vi "Autonomous Independent.vi"() -> ()   [LabVIEW 2015]
doc: "This VI is called when autonomous begins, and will automatically be terminated when autonomous ends. You can carry out timed or sensor driven robot movement independently without needing to return to the caller."
uses:
  Type Defs/Auto Defense.ctl
  Type Defs/Auto Goal.ctl
  Type Defs/Auto Position.ctl
  Type Defs/Auto Goal Drive P4 M.ctl
  Type Defs/Auto Rough Terrain Cross.ctl
  Robot Global Data.vi
  <vilib>/addons/control/pid/pid.llb/PID (DBL).vi
  Type Defs/Auto Porticullis cross.ctl
  Type Defs/Auto Chival Cross.ctl
  Type Defs/Auto goal drive P5 R.ctl
  <instrlib>/navX Library v2/navX Library v2.lvlib
  Type Defs/Auto Goal Drive P4 R.ctl
  <vilib>/addons/control/pid/NI_PID_pid.lvlib
panel:
  in  "3nd fwd distance":dbl=4.0 format="%#_13g"
  in  "3nd fwd speed":dbl=-0.8 format="%#_13g"
  in  "Adjust Deadband Cross":dbl=0.5
  in  "Range Adjust":cluster{"output high":dbl, "output low":dbl}={"output high"=0.8, "output low"=-0.8} {"output low" format="%.2f"; "output high" format="%.2f"}
  in  "PID Adjust":T1={"proportional gain (Kc)"=0.2, "integral time (Ti, min)"=0.01, "derivative time (Td, min)"=0.0} {"derivative time (Td, min)" format="%.3f"; "integral time (Ti, min)" format="%.3f"; "proportional gain (Kc)" format="%.3f"}
  out "Yaw":dbl
  in  "Angle Setpoint":dbl format="%.2f"
  in  "PID Port 2":T1={"proportional gain (Kc)"=0.2, "integral time (Ti, min)"=0.01, "derivative time (Td, min)"=0.0} {"derivative time (Td, min)" format="%.3f"; "integral time (Ti, min)" format="%.3f"; "proportional gain (Kc)" format="%.3f"}
  in  "Range Port 2":cluster{"output high":dbl, "output low":dbl}={"output high"=0.8, "output low"=-0.8} {"output low" format="%.2f"; "output high" format="%.2f"}
  in  "Port 1st speed 2":dbl=-0.7
  in  "Port 1st Distance 2":dbl=4.5 format="%#_13g"
  in  "1st Turn Speed":dbl format="%#_13g"
  in  "1st turn angle":dbl format="%#_13g"
  in  "2nd fwd distance":dbl=4.0 format="%#_13g"
  in  "2nd fwd speed":dbl=-0.8 format="%#_13g"
  in  "2nd turn angle":dbl=-70.0 format="%#_13g"
  in  "2nd Turn Speed":dbl=0.7 format="%#_13g"
  in  "1st fwd speed":dbl=-0.75 format="%#_13g"
  in  "1st fwd distance":dbl=10.0 format="%#_13g"
  in  "RT Adjust Deadband":dbl=3.0
  in  "Range RT":cluster{"output high":dbl, "output low":dbl}={"output high"=0.8, "output low"=-0.8} {"output low" format="%.2f"; "output high" format="%.2f"}
  in  "PID RT":T1={"proportional gain (Kc)"=0.08, "integral time (Ti, min)"=0.01, "derivative time (Td, min)"=0.0} {"derivative time (Td, min)" format="%.3f"; "integral time (Ti, min)" format="%.3f"; "proportional gain (Kc)" format="%.3f"}
  in  "RT 1st Distance":dbl=9.5 format="%#_13g"
  in  "RT 2nd Speed":dbl=-0.9 format="%#_13g"
  in  "RT 1st speed":dbl=-0.9
  in  "RT speed error":dbl format="%#_13g"
  in  "RT shift speed distance":dbl=3.0 format="%#_13g"
  in  "2nd Distance Speed":dbl=-0.9 format="%#_13g"
  in  "Range Port":cluster{"output high":dbl, "output low":dbl}={"output high"=0.8, "output low"=-0.8} {"output low" format="%.2f"; "output high" format="%.2f"}
  in  "PID Port":T1={"proportional gain (Kc)"=0.2, "integral time (Ti, min)"=0.01, "derivative time (Td, min)"=0.0} {"derivative time (Td, min)" format="%.3f"; "integral time (Ti, min)" format="%.3f"; "proportional gain (Kc)" format="%.3f"}
  in  "Port 1st Distance":dbl=4.5 format="%#_13g"
  in  "Left Adjust":dbl
  in  "Right Adjust speed":dbl
  in  "Left Adjust speed":dbl
  in  "1st Distance Speed":dbl=-0.75 format="%#_13g"
  in  "Distance 1 Goal":dbl=11.5 format="%#_13g"
  in  "Chival Adjust Deadband":dbl=0.5
  in  "Range Chival":cluster{"output high":dbl, "output low":dbl}={"output high"=0.8, "output low"=-0.8} {"output low" format="%.2f"; "output high" format="%.2f"}
  in  "PID Chival":T1={"proportional gain (Kc)"=0.2, "integral time (Ti, min)"=0.01, "derivative time (Td, min)"=0.0} {"derivative time (Td, min)" format="%.3f"; "integral time (Ti, min)" format="%.3f"; "proportional gain (Kc)" format="%.3f"}
  in  "Arm Lift Distance":dbl=1.7 format="%#_13g"
  in  "Chival 2nd distance":dbl=6.0 format="%#_13g"
  in  "Chival Speed 2":dbl=-0.7
  in  "Chival Arm":dbl=100.0 format="%#_13g"
  in  "Chival Distance 1":dbl=3.0 format="%#_13g"
  in  "Chival speed":dbl=-0.7
  in  "Port 1st speed":dbl=-0.7
  in  "Distancia 1":dbl=3.0 format="%#_13g"
  in  "speed error":dbl=0.07 format="%#_13g"
  in  "velocidade 1":dbl
  in  "Adjust speed":dbl=-0.6 format="%#_13g"
  out "encoder":dbl
  out "x >= y?":bool
  out "Auto Angle":dbl
  out "erro":dbl
  in  "velocidade 2":dbl=0.7 format="%#_13g"
  in  "distancia 2":dbl=5.0 format="%#_13g"
  out "YRPHfH":T2
  # "Go to Right Goal from pos 5"
  # "Go to Middle goal from pos 4"
  # "Chival"
  # "Port"
  # "F lenta\nT Rapida"
  # "Rought Terrain"
  # "ramparts\nD 11"
  # "distancia speed\nrock wall 12 -1\n moat"
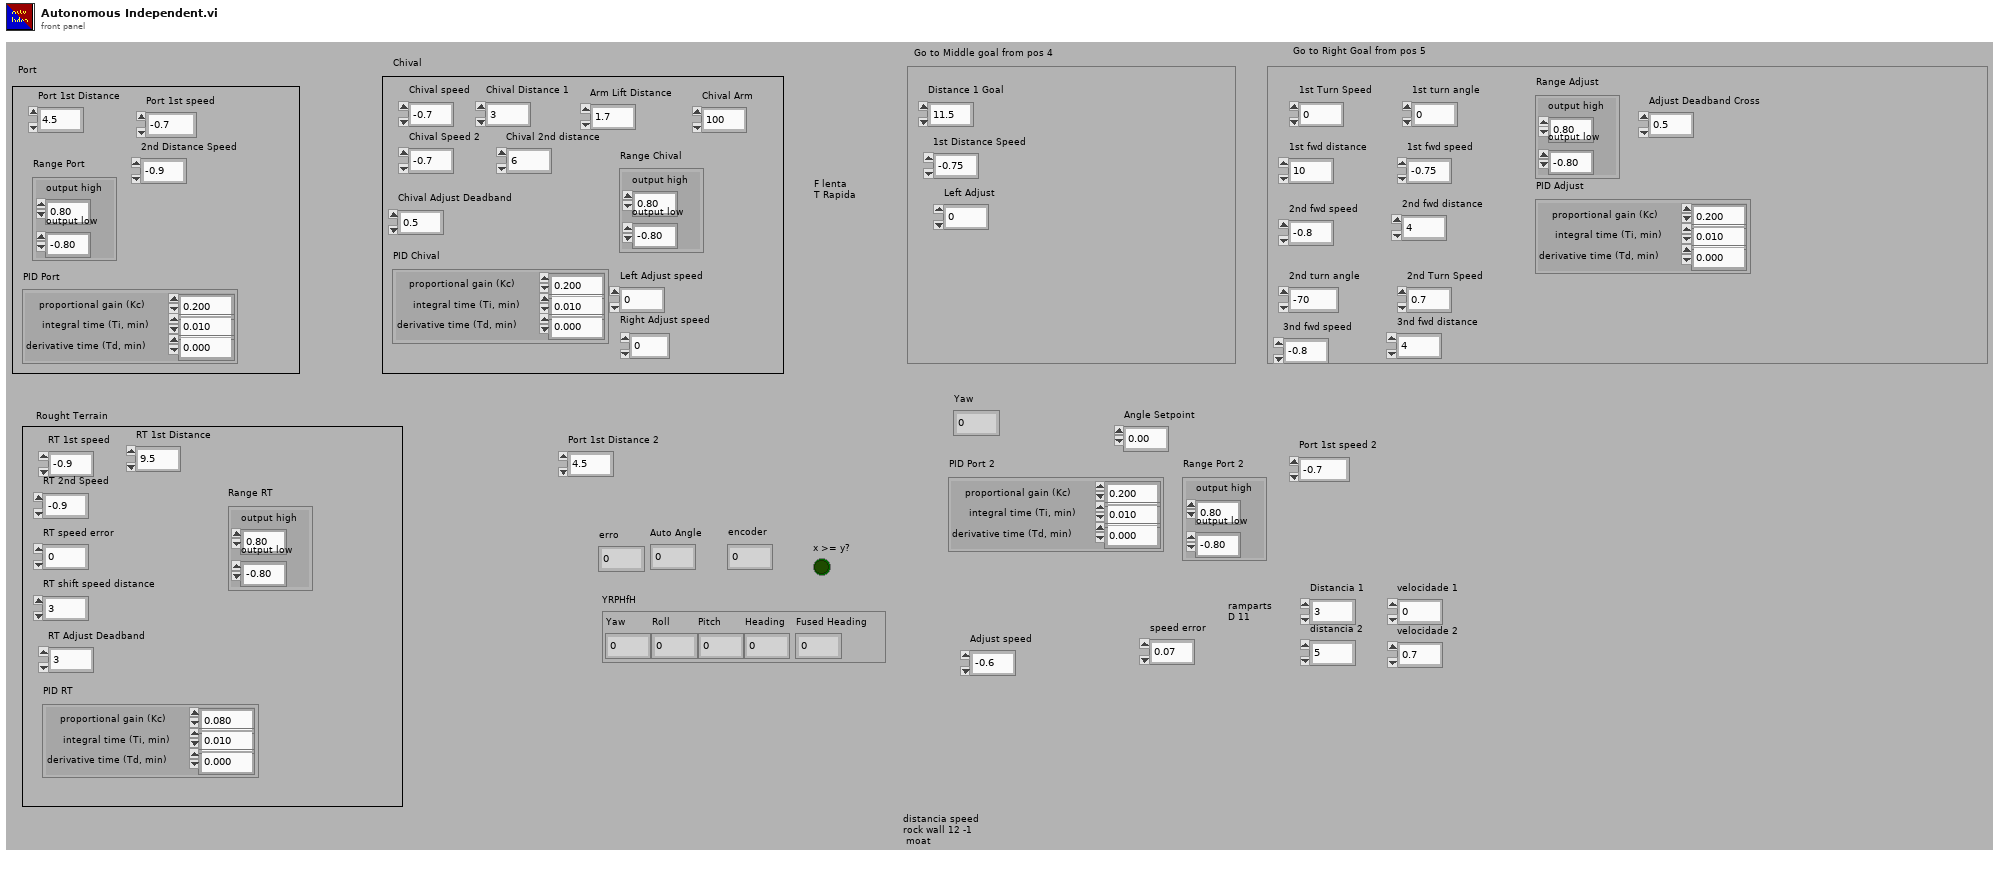
[diagram p1: front panel]
types:
  T1 = cluster{"proportional gain (Kc)":dbl, "integral time (Ti, min)":dbl, "derivative time (Td, min)":dbl}
  T2 = cluster{"Yaw":dbl, "Roll":dbl, "Pitch":dbl, "Heading":dbl, "Fused Heading":dbl}
  T3 = typedef "Auto Defense.ctl" = enum16{"Porticullis", "Chival de Frise", "Rough Terrain", "Rock Wall", "Ramparts", "Moat"}
  T4 = typedef "Auto Position.ctl" = enum16{"Pos 2", "Pos 3", "Pos 4", "Pos 5"}
  T5 = typedef "Auto Goal.ctl" = enum16{"Right Goal", "Left Goal", "Middle Goal"}
  T6 = typedef "Auto Goal Drive P4 R.ctl" = enum16{"Wait Defense Cross", "Turn Right", "Wait 1", "1st Forward", "Wait 2", "Turn Left", "Wait 3", "Adjust Left", "3rd Forward", "SHOOOOT", "Prepare Shoot"}
  T7 = typedef "Auto goal drive P5 R.ctl" = enum16{"Wait defense cross", "Adjust Right", "Wait 1", "1st Fwd", "Adjust Angle", "Wait 2", "2nd Fwd", "Turn Left", "Wait 3", "3nd Fwd", "Shoot"}
  T8 = typedef "Auto Goal Drive P4 M.ctl" = enum16{"Wait Defense Cross", "Prepare Shooter", "Go Fwd", "Shoot"}
  T9 = typedef "Auto Porticullis cross.ctl" = enum16{"Set Navx", "Go Fwd", "Wait 1", "Cross Porticullis", "Get Navx", "Adjust angle", "Wait 2", "Finish"}
  T10 = typedef "Auto Chival Cross.ctl" = enum16{"Set NavX", "Go Fwd", "Lower Arm", "Slow Fwd", "Get NavX", "Adjust Angle", "Wait", "Finish"}
  T11 = typedef "Auto Rough Terrain Cross.ctl" = enum16{"Set NavX", "Go Fwd", "Get Navx", "Correct Angle", "Wait", "Go to Goal"}
  T12 = enum16{"Set NavX", "Go Fwd", "Get Navx", "Correct Angle", "Go to Goal"}
  T13 = typedef "navX Library v2.lvlib/Z900_navX_DeviceTypeDef.ctl" = cluster{"Interface":cluster{"Protocol":T14, "Update Rate (4Hz-60Hz)":u8, "navX Open TypeDef":variant}, "Notify Packet":refnum<notifier>, "Loop VI Refnum":refnum<vi>, "Ready to Close Occurrence Refnum":refnum<k4>}
  T14 = typedef "navX Library v2.lvlib/Z900_navX_ProtocolTypeDef.ctl" = enum16{"SERIAL", "I2C", "SPI"}
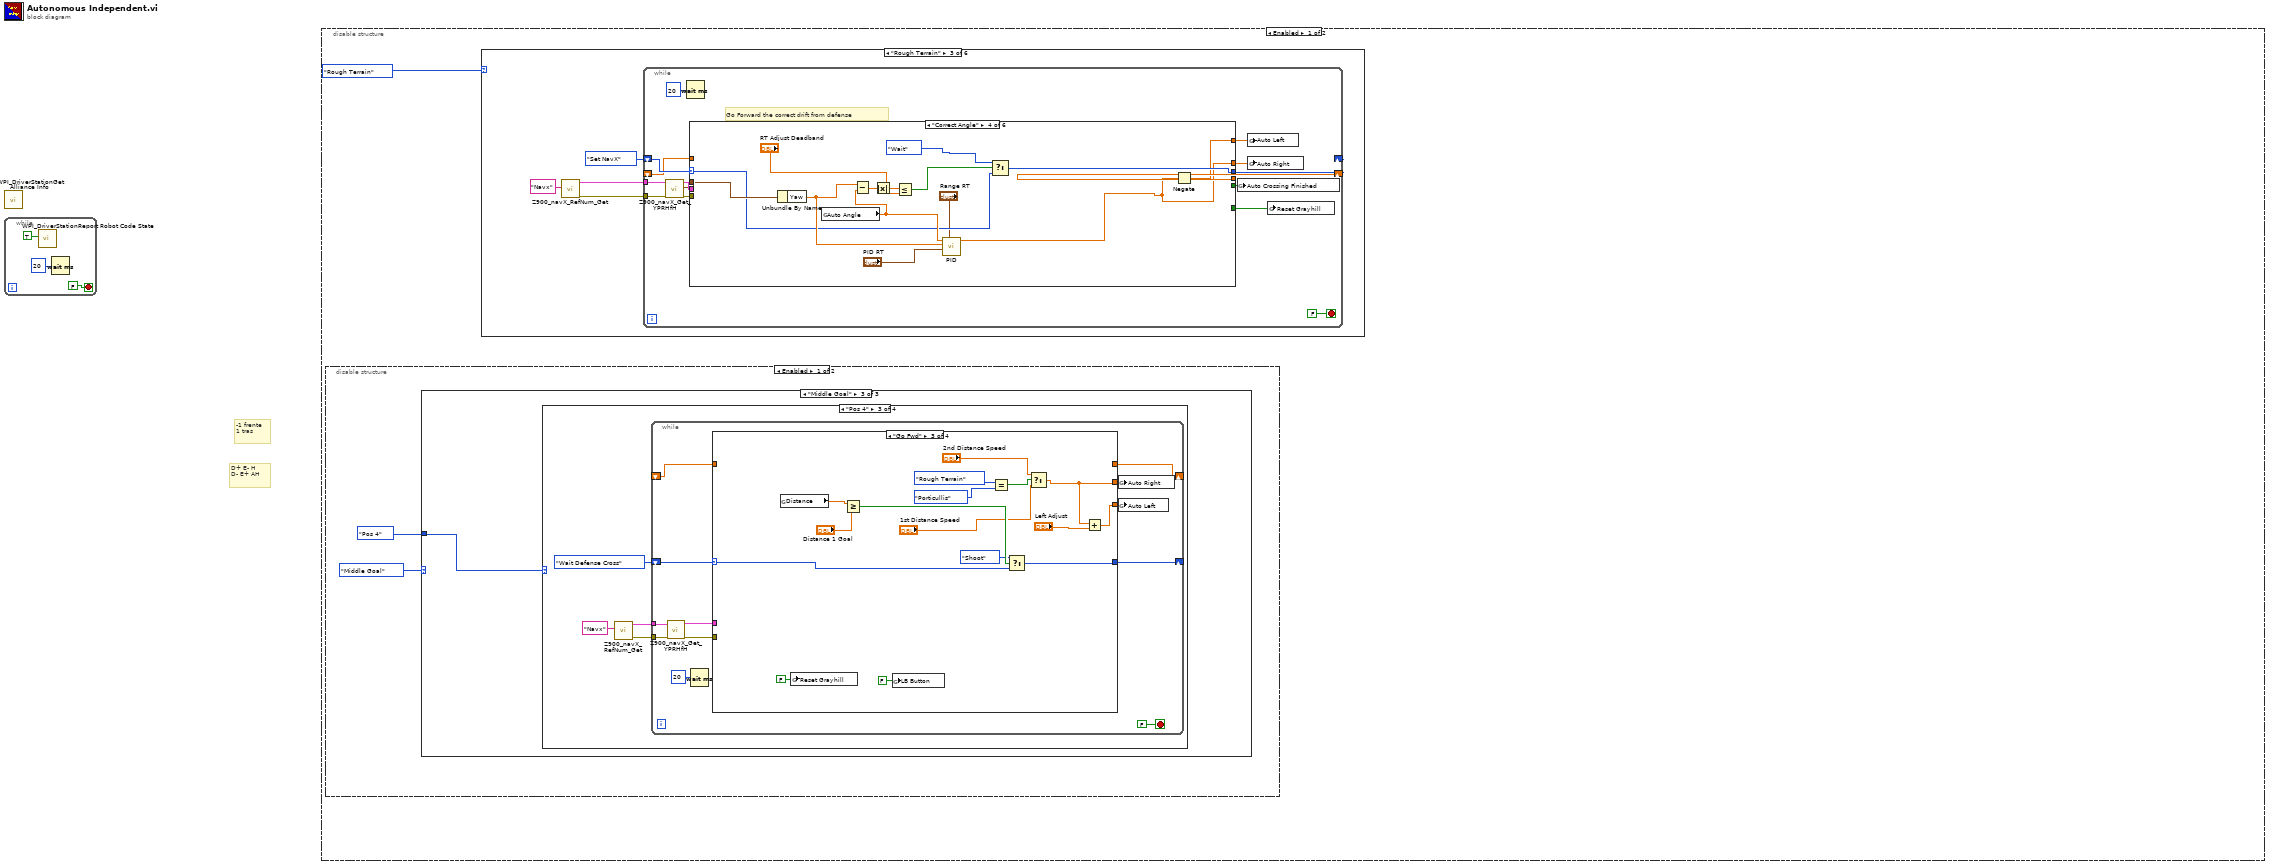
[diagram p0: block diagram]
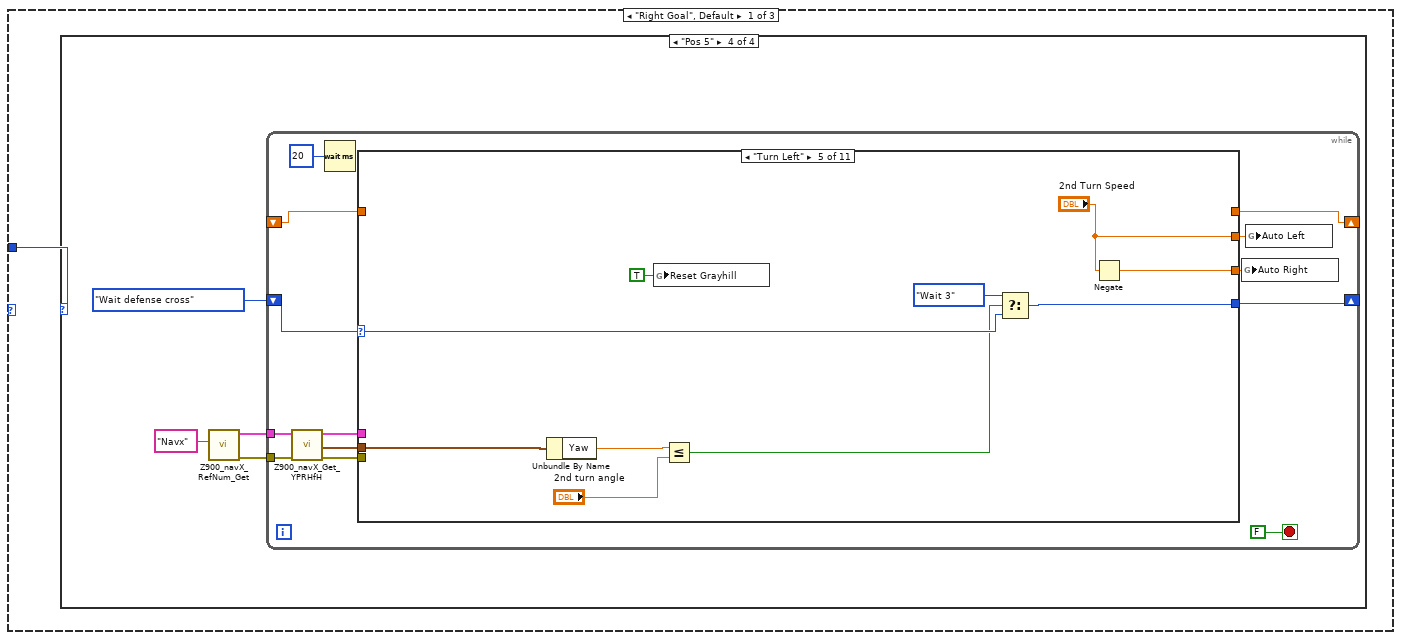
[diagram p2: hidden frame]
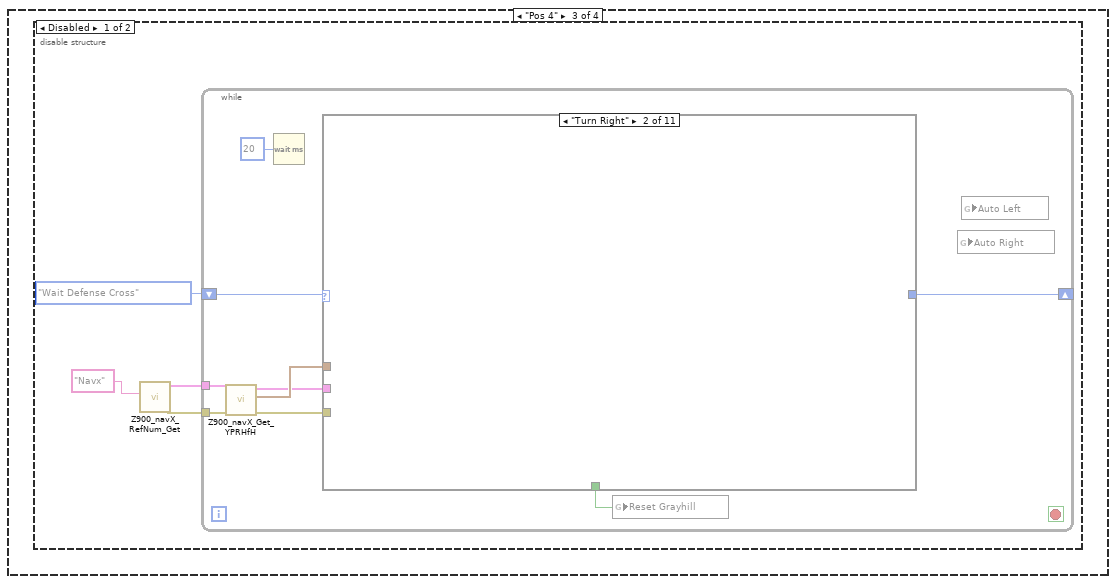
[diagram p5: hidden frame]
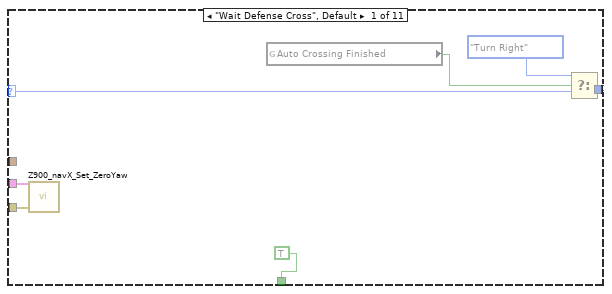
[diagram p6: hidden frame]
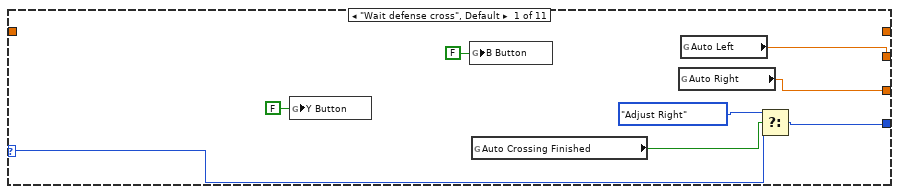
[diagram p17: hidden frame]
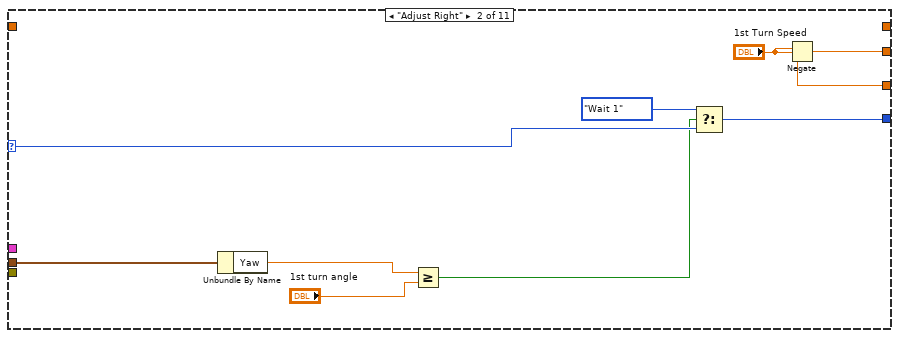
[diagram p18: hidden frame]
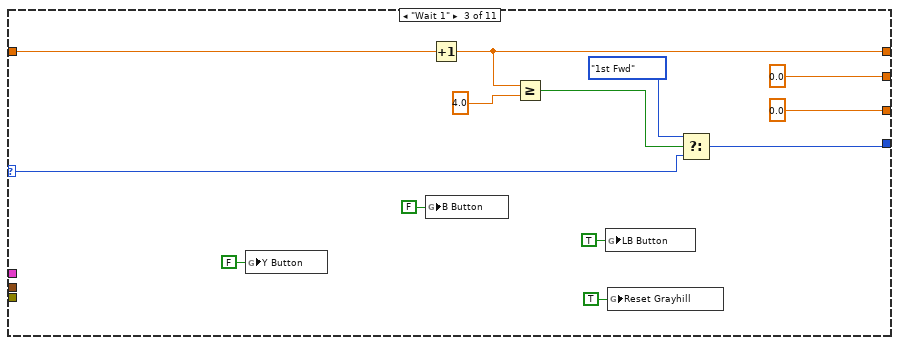
[diagram p19: hidden frame]
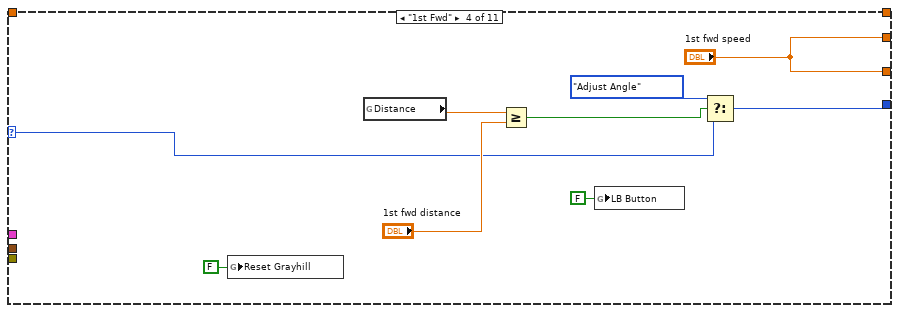
[diagram p20: hidden frame]
diagram:
  # "D+ E- H\nD- E+ AH"
  # "-1 frente\n1 tras"
  n1 = call <vilib>:"WPI_DriverStationGet Alliance Info.vi"() -> ()  [unwired: 12 out]
  n2 = while {
    stop <- FALSE stop-if-true
    n3 = call <vilib>:"WPI_DriverStationReport Robot Code State.vi"("Autonomous"=TRUE) -> ()  [unwired: 10 in, 1 out]
    n4 = Wait (ms)(milliseconds to wait=u32 20) -> ()  [unwired: 1 out]
  }
  n5 = disable-structure shown="Enabled" {
    frame Enabled {
      n6 = disable-structure shown="Enabled" {
        frame Enabled {
          n7 = case shown="\"Middle Goal\"" Auto_Goal."Middle Goal" {
            tunnel: Auto_Position."Pos 4" -> [w7 w150 w151]
            frame "Right Goal", Default {
              n8 = case shown="\"Pos 5\"" w7 {
                frame "Pos 2", Default {
                }
                frame "Pos 3" {
                }
                frame "Pos 4" {
                  n9 = disable-structure shown="Disabled" {
                    frame Disabled {
                      n10 = call <instrlib>:"Z900_navX_RefNum_Get.vi"("refnum name"="Navx") -> ("error out"=w8:errorcluster, "navX Device"=w9:T13)  [unwired: 9 in]
                      n11 = while {
                        shift-right: [w14] -> _
                        shift-left: Auto_Goal_Drive_P4_R."Wait Defense Cross" -> [w20]
                        tunnel: w9 -> [w19]
                        tunnel: w8 -> [w18]
                        stop <- _ stop-if-true
                        n12 = call <instrlib>:"Z900_navX_Get_YPRHfH.vi"("error in (no error)"=w18, "navX Device"=w19) -> ("error out"=w15:errorcluster, "YRPHfH"=w17:T2, "navX Device"=w16:T13)  [unwired: 6 in, 1 out]
                        n13 = Wait (ms)(milliseconds to wait=u32 20) -> ()  [unwired: 1 out]
                        n14 = case shown="\"Turn Right\"" w20 {
                          selector: w20 -> [w24 _ _ _ _ _ _ _ _ _ _]
                          tunnel: w17 -> [_ _ _ _ _ _ _ _ _ _ _]
                          tunnel: w16 -> [w27 _ _ _ _ _ _ _ _ _ _]
                          tunnel: w15 -> [w26 _ _ _ _ _ _ _ _ _ _]
                          tunnel: [w25 _ _ _ _ _ _ _ _ _ _] -> w14
                          tunnel: [TRUE _ _ _ _ _ _ _ _ _ _] -> w12
                          frame "Wait Defense Cross", Default {
                            n15 = call <instrlib>:"Z900_navX_Set_ZeroYaw.vi"("error in (no error)"=w26, "navX Device"=w27) -> ()  [unwired: 8 in, 2 out]
                            n16 = global read "Robot Global Data.vi" "Auto Crossing Finished"() -> (w22:bool)
                            n17 = Select(t=Auto_Goal_Drive_P4_R."Turn Right", s=w22, f=w24) -> (s? t:f=w25:T6)
                          }
                          frame "Turn Right" {
                          }
                          frame "Wait 1" {
                          }
                          frame "1st Forward" {
                          }
                          frame "Wait 2" {
                          }
                          frame "Turn Left" {
                          }
                          frame "Wait 3" {
                          }
                          frame "Adjust Left" {
                          }
                          frame "3rd Forward" {
                          }
                          frame "SHOOOOT" {
                          }
                          frame "Prepare Shoot" {
                          }
                        }
                        n18 = global write "Robot Global Data.vi" "Reset Grayhill"(w12) -> ()
                        n19 = global read "Robot Global Data.vi" "Auto Right"() -> ()  [unwired: 1 in]
                        n20 = global read "Robot Global Data.vi" "Auto Left"() -> ()  [unwired: 1 in]
                      }
                    }
                    frame Enabled {
                    }
                  }
                }
                frame "Pos 5" {
                  n21 = call <instrlib>:"Z900_navX_RefNum_Get.vi"("refnum name"="Navx") -> ("error out"=w28:errorcluster, "navX Device"=w29:T13)  [unwired: 9 in]
                  n22 = while {
                    shift-right: [w42] -> _
                    shift-left: Auto_goal_drive_P5_R."Wait defense cross" -> [w44]
                    tunnel: w29 -> [w40]
                    tunnel: w28 -> [w39]
                    shift-right: [w32] -> _
                    shift-left: _ -> [w33]
                    stop <- FALSE stop-if-true
                    n23 = call <instrlib>:"Z900_navX_Get_YPRHfH.vi"("error in (no error)"=w39, "navX Device"=w40) -> ("error out"=w34:errorcluster, "YRPHfH"=w38:T2, "navX Device"=w35:T13)  [unwired: 6 in, 1 out]
                    n24 = Wait (ms)(milliseconds to wait=u32 20) -> ()  [unwired: 1 out]
                    n25 = case shown="\"Turn Left\"" w44 {
                      selector: w44 -> [w51 w59 w70 w76 w92 _ w103 w112 w119 w131 w145]
                      tunnel: [w52 w60 w71 w78 w93 Auto_goal_drive_P5_R."Shoot" w104 w114 w120 w130 w144] -> w42
                      tunnel: w38 -> [_ w61 _ _ w91 _ _ _ _ w132 _]
                      tunnel: [w48 w54 0.0 "1st fwd speed" "2nd Turn Speed" w99 "2nd fwd speed" 0.0 "3nd fwd speed" w128 0.0] -> w37
                      tunnel: [w47 "1st Turn Speed" 0.0 "1st fwd speed" w85 w99 "2nd fwd speed" 0.0 "3nd fwd speed" w127 0.0] -> w36
                      tunnel: w35 -> [_ _ _ _ _ _ _ _ _ _ _]
                      tunnel: w34 -> [_ _ _ _ _ _ _ _ _ _ _]
                      tunnel: w33 -> [_ _ w69 _ _ w97 _ w111 _ _ w146]
                      tunnel: [_ _ w68 _ _ w96 _ w113 _ _ w141] -> w32
                      frame "Wait defense cross", Default {
                        n26 = global write "Robot Global Data.vi" "Y Button"(FALSE ("Y Button")) -> ()
                        n27 = global write "Robot Global Data.vi" "B Button"(FALSE ("B Button")) -> ()
                        n28 = global read "Robot Global Data.vi" "Auto Crossing Finished"() -> (w49:bool)
                        n29 = global read "Robot Global Data.vi" "Auto Right"() -> (w47:dbl)
                        n30 = global read "Robot Global Data.vi" "Auto Left"() -> (w48:dbl)
                        n31 = Select(t=Auto_goal_drive_P5_R."Adjust Right", s=w49, f=w51) -> (s? t:f=w52:T7)
                      }
                      frame "Adjust Right" {
                        n32 = Unbundle By Name(w61) -> ("Yaw"=w58:dbl)
                        n33 = Greater Or Equal?(x=w58, y="1st turn angle") -> (x >= y?=w56:bool)
                        n34 = Select(t=Auto_goal_drive_P5_R."Wait 1", s=w56, f=w59) -> (s? t:f=w60:T7)
                        n35 = Negate(x="1st Turn Speed") -> (-x=w54:dbl)
                      }
                      frame "Wait 1" {
                        n36 = global write "Robot Global Data.vi" "Y Button"(FALSE ("Y Button")) -> ()
                        n37 = global write "Robot Global Data.vi" "B Button"(FALSE ("B Button")) -> ()
                        n38 = Increment(x=w69) -> (x+1=w68:dbl)
                        n39 = Greater Or Equal?(x=w68, y=4.0) -> (x >= y?=w67:bool)
                        n40 = global write "Robot Global Data.vi" "LB Button"(TRUE ("LB Button")) -> ()
                        n41 = global write "Robot Global Data.vi" "Reset Grayhill"(TRUE ("Reset Grayhill")) -> ()
                        n42 = Select(t=Auto_goal_drive_P5_R."1st Fwd", s=w67, f=w70) -> (s? t:f=w71:T7)
                      }
                      frame "1st Fwd" {
                        n43 = global write "Robot Global Data.vi" "Reset Grayhill"(FALSE ("Reset Grayhill")) -> ()
                        n44 = global read "Robot Global Data.vi" "Distance"() -> (w80:dbl)
                        n45 = Greater Or Equal?(x=w80, y="1st fwd distance") -> (x >= y?=w77:bool)
                        n46 = global write "Robot Global Data.vi" "LB Button"(FALSE ("LB Button")) -> ()
                        n47 = Select(t=Auto_goal_drive_P5_R."Adjust Angle", s=w77, f=w76) -> (s? t:f=w78:T7)
                      }
                      frame "Turn Left" {
                        n48 = Unbundle By Name(w91) -> ("Yaw"=w89:dbl)
                        n49 = global write "Robot Global Data.vi" "Reset Grayhill"(TRUE ("Reset Grayhill")) -> ()
                        n50 = Less Or Equal?(x=w89, y="2nd turn angle") -> (x <= y?=w87:bool)
                        n51 = Select(t=Auto_goal_drive_P5_R."Wait 3", s=w87, f=w92) -> (s? t:f=w93:T7)
                        n52 = Negate(x="2nd Turn Speed") -> (-x=w85:dbl)
                      }
                      frame "Shoot" {
                        w99 = -0.3
                        n53 = Increment(x=w97) -> (x+1=w96:dbl)
                        n54 = Greater Or Equal?(x=w96, y=20.0) -> (x >= y?=w94:bool)
                        n55 = global write "Robot Global Data.vi" "RB Trigger"(w94) -> ()
                      }
                      frame "2nd Fwd" {
                        n56 = global read "Robot Global Data.vi" "Distance"() -> (w107:dbl)
                        n57 = Greater Or Equal?(x=w107, y="2nd fwd distance") -> (x >= y?=w102:bool)
                        n58 = global write "Robot Global Data.vi" "Reset Grayhill"(FALSE ("Reset Grayhill")) -> ()
                        n59 = Select(t=Auto_goal_drive_P5_R."Turn Left", s=w102, f=w103) -> (s? t:f=w104:T7)
                      }
                      frame "Wait 3" {
                        n60 = Increment(x=w111) -> (x+1=w113:dbl)
                        n61 = Greater Or Equal?(x=w113, y=4.0) -> (x >= y?=w117:bool)
                        n62 = global write "Robot Global Data.vi" "Reset Grayhill"(TRUE ("Reset Grayhill")) -> ()
                        n63 = Select(t=Auto_goal_drive_P5_R."3nd Fwd", s=w117, f=w112) -> (s? t:f=w114:T7)
                      }
                      frame "3nd Fwd" {
                        n64 = global read "Robot Global Data.vi" "Distance"() -> (w125:dbl)
                        n65 = Greater Or Equal?(x=w125, y="3nd fwd distance") -> (x >= y?=w123:bool)
                        n66 = Select(t=Auto_goal_drive_P5_R."Shoot", s=w123, f=w119) -> (s? t:f=w120:T7)
                        n67 = global write "Robot Global Data.vi" "Reset Grayhill"(FALSE ("Reset Grayhill")) -> ()
                      }
                      frame "Adjust Angle" {
                        n68 = Unbundle By Name(w132) -> ("Yaw"=w138:dbl)
                        n69 = global read "Robot Global Data.vi" "Auto Angle"() -> (w137:dbl)
                        n70 = Subtract(x=w138, y=w137) -> (x-y=w136:dbl)
                        n71 = Absolute Value(x=w136) -> (abs(x)=w135:dbl)
                        n72 = Less Or Equal?(x=w135, y="Adjust Deadband Cross") -> (x <= y?=w133:bool)
                        n73 = call-poly <vilib>:"PID.vi"("output range"="Range Adjust", "PID gains"="PID Adjust", "process variable"=w138, "setpoint"=w137) -> ("output"=w127:dbl)  [unwired: 6 in, 1 out]
                        n74 = Select(t=Auto_goal_drive_P5_R."Wait 2", s=w133, f=w131) -> (s? t:f=w130:T7)
                        n75 = Negate(x=w127) -> (-x=w128:dbl)
                      }
                      frame "Wait 2" {
                        n76 = global write "Robot Global Data.vi" "Reset Grayhill"(TRUE ("Reset Grayhill")) -> ()
                        n77 = Increment(x=w146) -> (x+1=w141:dbl)
                        n78 = Greater Or Equal?(x=w141, y=4.0) -> (x >= y?=w149:bool)
                        n79 = Select(t=Auto_goal_drive_P5_R."2nd Fwd", s=w149, f=w145) -> (s? t:f=w144:T7)
                      }
                    }
                    n80 = global write "Robot Global Data.vi" "Auto Right"(w36) -> ()
                    n81 = global write "Robot Global Data.vi" "Auto Left"(w37) -> ()
                  }
                }
              }
            }
            frame "Left Goal" {
              n82 = case shown="\"Pos 3\"" w150 {
                frame "Pos 2", Default {
                }
                frame "Pos 3" {
                }
                frame "Pos 4" {
                }
                frame "Pos 5" {
                }
              }
            }
            frame "Middle Goal" {
              n83 = case shown="\"Pos 4\"" w151 {
                frame "Pos 2", Default {
                }
                frame "Pos 3" {
                }
                frame "Pos 4" {
                  n84 = call <instrlib>:"Z900_navX_RefNum_Get.vi"("refnum name"="Navx") -> ("error out"=w152:errorcluster, "navX Device"=w153:T13)  [unwired: 9 in]
                  n85 = while {
                    shift-right: [w164] -> _
                    shift-left: Auto_Goal_Drive_P4_M."Wait Defense Cross" -> [w167]
                    tunnel: w153 -> [w163]
                    tunnel: w152 -> [w162]
                    shift-right: [w157] -> _
                    shift-left: _ -> [w156]
                    stop <- FALSE stop-if-true
                    n86 = call <instrlib>:"Z900_navX_Get_YPRHfH.vi"("error in (no error)"=w162, "navX Device"=w163) -> ("error out"=w160:errorcluster, "navX Device"=w161:T13)  [unwired: 6 in, 2 out]
                    n87 = Wait (ms)(milliseconds to wait=u32 20) -> ()  [unwired: 1 out]
                    n88 = case shown="\"Go Fwd\"" w167 {
                      selector: w167 -> [w173 w176 w197 _]
                      tunnel: [w172 w177 w198 Auto_Goal_Drive_P4_M."Shoot"] -> w164
                      tunnel: w161 -> [_ _ _ _]
                      tunnel: w160 -> [_ _ _ _]
                      tunnel: [w170 w182 w191 w208] -> w159
                      tunnel: [w169 w182 w188 w208] -> w158
                      tunnel: [_ w180 _ w210] -> w157
                      tunnel: w156 -> [_ w181 _ w211]
                      frame "Wait Defense Cross", Default {
                        w168 = FALSE
                        n89 = global read "Robot Global Data.vi" "Auto Crossing Finished"() -> (w174:bool)
                        n90 = global write "Robot Global Data.vi" "B Button"(w168) -> ()
                        n91 = global write "Robot Global Data.vi" "Y Button"(w168) -> ()
                        n92 = Select(t=Auto_Goal_Drive_P4_M."Prepare Shooter", s=w174, f=w173) -> (s? t:f=w172:T8)
                        n93 = global read "Robot Global Data.vi" "Auto Right"() -> (w169:dbl)
                        n94 = global read "Robot Global Data.vi" "Auto Left"() -> (w170:dbl)
                      }
                      frame "Prepare Shooter" {
                        w182 = 0.0 ("Auto Right")
                        n95 = global write "Robot Global Data.vi" "Reset Grayhill"(TRUE ("Reset Grayhill")) -> ()
                        n96 = Increment(x=w181) -> (x+1=w180:dbl)
                        n97 = global write "Robot Global Data.vi" "LB Button"(TRUE ("LB Button")) -> ()
                        n98 = Greater Or Equal?(x=w180, y=5.0) -> (x >= y?=w175:bool)
                        n99 = Select(t=Auto_Goal_Drive_P4_M."Go Fwd", s=w175, f=w176) -> (s? t:f=w177:T8)
                      }
                      frame "Go Fwd" {
                        n100 = global read "Robot Global Data.vi" "Distance"() -> (w196:dbl)
                        n101 = global write "Robot Global Data.vi" "Reset Grayhill"(FALSE ("Reset Grayhill")) -> ()
                        n102 = Greater Or Equal?(x=w196, y="Distance 1 Goal") -> (x >= y?=w194:bool)
                        n103 = global write "Robot Global Data.vi" "LB Button"(FALSE ("LB Button")) -> ()
                        n104 = Equal?(x=Auto_Defense."Rough Terrain", y=Auto_Defense."Porticullis") -> (x = y?=w187:bool)
                        n105 = Select(t=Auto_Goal_Drive_P4_M."Shoot", s=w194, f=w197) -> (s? t:f=w198:T8)
                        n106 = Select(t="2nd Distance Speed", s=w187, f="1st Distance Speed") -> (s? t:f=w188:dbl)
                        n107 = Add(x=w188, y="Left Adjust") -> (x+y=w191:dbl)
                      }
                      frame "Shoot" {
                        w208 = -0.6 ("Auto Right")
                        # "Alterar para chamada da dashboard"
                        n108 = Increment(x=w211) -> (x+1=w210:dbl)
                        n109 = Equal?(x=Auto_Defense."Rough Terrain", y=Auto_Defense."Porticullis") -> (x = y?=w203:bool)
                        n110 = Select(t=80.0 ("y"), s=w203, f=40.0) -> (s? t:f=w204:dbl)
                        n111 = Greater Or Equal?(x=w210, y=w204) -> (x >= y?=w207:bool)
                        n112 = global write "Robot Global Data.vi" "RB Trigger"(w207) -> ()
                      }
                    }
                    n113 = global write "Robot Global Data.vi" "Auto Right"(w158) -> ()
                    n114 = global write "Robot Global Data.vi" "Auto Left"(w159) -> ()
                  }
                }
                frame "Pos 5" {
                }
              }
            }
          }
        }
        frame Disabled {
        }
      }
      n115 = case shown="\"Rough Terrain\"" Auto_Defense."Rough Terrain" {
        frame "Porticullis", Default {
          n116 = disable-structure shown="Enabled" {
            frame Enabled {
              n117 = call <instrlib>:"Z900_navX_RefNum_Get.vi"("refnum name"="Navx") -> ("error out"=w213:errorcluster, "navX Device"=w214:T13)  [unwired: 9 in]
              n118 = while {
                shift-right: [w231] -> _
                shift-left: Auto_Porticullis_cross."Set Navx" -> [w232]
                tunnel: w214 -> [w230]
                tunnel: w213 -> [w229]
                shift-right: [w225] -> _
                shift-left: _ -> [w224]
                shift-right: [w216] -> _
                shift-left: _ -> [w217]
                stop <- FALSE stop-if-true
                n119 = call <instrlib>:"Z900_navX_Get_YPRHfH.vi"("error in (no error)"=w229, "navX Device"=w230) -> ("error out"=w228:errorcluster, "YRPHfH"=w226:T2, "navX Device"=w227:T13)  [unwired: 6 in, 1 out]
                n120 = Wait (ms)(milliseconds to wait=u32 20) -> ()  [unwired: 1 out]
                n121 = case shown="\"Set Navx\", Default" w232 {
                  selector: w232 -> [w241 w248 w257 w268 w277 w291 _ w308]
                  tunnel: [w242 w250 w258 w269 w276 w290 Auto_Porticullis_cross."Finish" w310] -> w231
                  tunnel: w228 -> [w240 _ _ _ _ _ _ _]
                  tunnel: w227 -> [w239 _ _ _ _ _ _ _]
                  tunnel: w226 -> [w238 _ _ _ w278 w292 _ _]
                  tunnel: [w237 _ w259 _ w279 _ _ _] -> w225
                  tunnel: w224 -> [w236 _ w264 _ w280 _ _ _]
                  tunnel: [w235 "Port 1st speed" 0.0 ("Port speed") 0.0 ("Port speed") w274 w286 w301 w312] -> w223
                  tunnel: [w235 "Port 1st speed" 0.0 ("Port speed") 0.0 ("Port speed") w274 w287 w302 w312] -> w222
                  tunnel: [TRUE _ TRUE w265 TRUE _ w300 _] -> w221
                  tunnel: [_ _ _ _ _ _ TRUE _] -> w219
                  tunnel: w217 -> [_ _ _ _ _ _ _ w311]
                  tunnel: [_ _ _ _ _ _ _ w307] -> w216
                  frame "Set Navx", Default {
                    w235 = 0.0
                    n122 = call <instrlib>:"Z900_navX_Set_ZeroYaw.vi"("error in (no error)"=w240, "navX Device"=w239) -> ()  [unwired: 8 in, 2 out]
                    n123 = Unbundle By Name(w238) -> ("Yaw"=w245:dbl)
                    n124 = Increment(x=w236) -> (x+1=w237:dbl)
                    n125 = global write "Robot Global Data.vi" "Auto Angle"(w245) -> ()
                    n126 = Greater Or Equal?(x=w237, y=3.0) -> (x >= y?=w243:bool)
                    n127 = Select(t=Auto_Porticullis_cross."Go Fwd", s=w243, f=w241) -> (s? t:f=w242:T9)
                  }
                  frame "Go Fwd" {
                    n128 = global write "Robot Global Data.vi" "B Button"(TRUE ("B Button")) -> ()
                    n129 = global read "Robot Global Data.vi" "Distance"() -> (w252:dbl)
                    n130 = Greater Or Equal?(x=w252, y="Port 1st Distance") -> (x >= y?=w249:bool)
                    n131 = Select(t=Auto_Porticullis_cross."Cross Porticullis", s=w249, f=w248) -> (s? t:f=w250:T9)
                  }
                  frame "Wait 1" {
                    n132 = global write "Robot Global Data.vi" "B Button"(FALSE ("B Button")) -> ()
                    n133 = Increment(x=w264) -> (x+1=w259:dbl)
                    n134 = Greater Or Equal?(x=w259, y=30.0) -> (x >= y?=w260:bool)
                    n135 = Select(t=Auto_Porticullis_cross."Cross Porticullis", s=w260, f=w257) -> (s? t:f=w258:T9)
                  }
                  frame "Cross Porticullis" {
                    n136 = global write "Robot Global Data.vi" "Start Button"(TRUE ("Start Button")) -> ()
                    n137 = global read "Robot Global Data.vi" "Finished Porticullis crossing"() -> (w267:bool)
                    n138 = Select(t=Auto_Porticullis_cross."Get Navx", s=w267, f=w268) -> (s? t:f=w269:T9)
                    n139 = global read "Robot Global Data.vi" "Reset Grayhill"() -> (w265:bool)
                  }
                  frame "Get Navx" {
                    w274 = 0.0
                    n140 = Unbundle By Name(w278) -> ("Yaw"=w285:dbl)
                    n141 = global read "Robot Global Data.vi" "Auto Angle"() -> (w284:dbl)
                    n142 = Increment(x=w280) -> (x+1=w279:dbl)
                    n143 = Greater Or Equal?(x=w279, y=3.0) -> (x >= y?=w281:bool)
                    n144 = Subtract(x=w285, y=w284) -> (x-y=w282:dbl)
                    n145 = Select(t=Auto_Porticullis_cross."Adjust angle", s=w281, f=w277) -> (s? t:f=w276:T9)
                    n146 = global write "Robot Global Data.vi" "Auto Angle error"(w282) -> ()
                  }
                  frame "Adjust angle" {
                    n147 = Unbundle By Name(w292) -> ("Yaw"=w297:dbl)
                    n148 = global read "Robot Global Data.vi" "Auto Angle"() -> (w296:dbl)
                    n149 = Subtract(x=w297, y=w296) -> (x-y=w295:dbl)
                    n150 = Absolute Value(x=w295) -> (abs(x)=w294:dbl)
                    n151 = Less Or Equal?(x=w294, y=3.0) -> (x <= y?=w293:bool)
                    n152 = call-poly <vilib>:"PID.vi"("output range"="Range Port", "PID gains"="PID Port", "process variable"=w297, "setpoint"=w296) -> ("output"=w287:dbl)  [unwired: 6 in, 1 out]
                    n153 = Select(t=Auto_Porticullis_cross."Wait 2", s=w293, f=w291) -> (s? t:f=w290:T9)
                    n154 = Negate(x=w287) -> (-x=w286:dbl)
                  }
                  frame "Finish" {
                    n155 = global read "Robot Global Data.vi" "Reset Grayhill"() -> (w300:bool)
                    n156 = global read "Robot Global Data.vi" "Auto Right"() -> (w302:dbl)
                    n157 = global read "Robot Global Data.vi" "Auto Left"() -> (w301:dbl)
                  }
                  frame "Wait 2" {
                    w312 = 0.0 ("Auto Right")
                    n158 = Increment(x=w311) -> (x+1=w307:dbl)
                    n159 = Greater Or Equal?(x=w307, y=25.0) -> (x >= y?=w305:bool)
                    n160 = Select(t=Auto_Porticullis_cross."Finish", s=w305, f=w308) -> (s? t:f=w310:T9)
                  }
                }
                n161 = global write "Robot Global Data.vi" "Auto Right"(w222) -> ()
                n162 = global write "Robot Global Data.vi" "Auto Left"(w223) -> ()
                n163 = global write "Robot Global Data.vi" "Reset Grayhill"(w221) -> ()
                n164 = global write "Robot Global Data.vi" "Auto Crossing Finished"(w219) -> ()
              }
            }
            frame Disabled {
            }
          }
        }
        frame "Chival de Frise" {
          n165 = call <instrlib>:"Z900_navX_RefNum_Get.vi"("refnum name"="Navx") -> ("error out"=w315:errorcluster, "navX Device"=w316:T13)  [unwired: 9 in]
          n166 = while {
            shift-right: [w334] -> _
            shift-left: Auto_Chival_Cross."Set NavX" -> [w335]
            tunnel: w316 -> [w333]
            tunnel: w315 -> [w332]
            shift-right: [w328] -> _
            shift-left: _ -> [w327]
            stop <- FALSE stop-if-true
            n167 = call <instrlib>:"Z900_navX_Get_YPRHfH.vi"("error in (no error)"=w332, "navX Device"=w333) -> ("error out"=w331:errorcluster, "YRPHfH"=w329:T2, "navX Device"=w330:T13)  [unwired: 6 in, 1 out]
            n168 = Wait (ms)(milliseconds to wait=u32 20) -> ()  [unwired: 1 out]
            n169 = case shown="\"Go Fwd\"" w335 {
              selector: w335 -> [w344 w350 w361 w373 w388 _ w399 w410]
              tunnel: [w345 w352 w362 w374 w387 Auto_Chival_Cross."Finish" w398 w411] -> w334
              tunnel: w331 -> [w343 _ _ _ _ _ _ _]
              tunnel: w330 -> [w342 _ _ _ _ _ _ _]
              tunnel: w329 -> [w341 _ _ _ w389 _ w400 _]
              tunnel: [w340 _ _ _ _ _ w401 w412] -> w328
              tunnel: w327 -> [w339 _ _ _ _ _ w402 w415]
              tunnel: [w338 "Chival speed" 0.0 ("Port speed") "Chival Speed 2" w377 w391 w396 w408] -> w322
              tunnel: [w338 "Chival speed" 0.0 ("Port speed") "Chival Speed 2" w376 w392 w396 w408] -> w319
              tunnel: [TRUE _ TRUE _ _ w390 TRUE _] -> w326
              tunnel: [_ _ _ _ _ TRUE _ _] -> w324
              frame "Set NavX", Default {
                w338 = 0.0
                n170 = call <instrlib>:"Z900_navX_Set_ZeroYaw.vi"("error in (no error)"=w343, "navX Device"=w342) -> ()  [unwired: 8 in, 2 out]
                n171 = Unbundle By Name(w341) -> ("Yaw"=w348:dbl)
                n172 = Increment(x=w339) -> (x+1=w340:dbl)
                n173 = global write "Robot Global Data.vi" "Auto Angle"(w348) -> ()
                n174 = Greater Or Equal?(x=w340, y=5.0) -> (x >= y?=w346:bool)
                n175 = Select(t=Auto_Chival_Cross."Go Fwd", s=w346, f=w344) -> (s? t:f=w345:T10)
              }
              frame "Go Fwd" {
                n176 = global read "Robot Global Data.vi" "Distance"() -> (w354:dbl)
                n177 = Greater Or Equal?(x=w354, y="Chival Distance 1") -> (x >= y?=w351:bool)
                n178 = Select(t=Auto_Chival_Cross."Lower Arm", s=w351, f=w350) -> (s? t:f=w352:T10)
              }
              frame "Lower Arm" {
                n179 = global write "Robot Global Data.vi" "B Button"(TRUE ("B Button")) -> ()
                n180 = global read "Robot Global Data.vi" "Arm Current Position"() -> (w358:dbl)
                n181 = Greater Or Equal?(x=w358, y="Chival Arm") -> (x >= y?=w356:bool)
                n182 = Select(t=Auto_Chival_Cross."Slow Fwd", s=w356, f=w361) -> (s? t:f=w362:T10)
              }
              frame "Slow Fwd" {
                n183 = global read "Robot Global Data.vi" "Distance"() -> (w369:dbl)
                n184 = global write "Robot Global Data.vi" "B Button"(FALSE ("Start Button")) -> ()
                n185 = Greater Or Equal?(x=w369, y="Chival 2nd distance") -> (x >= y?=w371:bool)
                n186 = Greater Or Equal?(x=w369, y="Arm Lift Distance") -> (x >= y?=w367:bool)
                n187 = Select(t=Auto_Chival_Cross."Get NavX", s=w371, f=w373) -> (s? t:f=w374:T10)
                n188 = global write "Robot Global Data.vi" "Y Button"(w367) -> ()
              }
              frame "Adjust Angle" {
                n189 = Unbundle By Name(w389) -> ("Yaw"=w383:dbl)
                n190 = global read "Robot Global Data.vi" "Auto Angle"() -> (w382:dbl)
                n191 = Subtract(x=w383, y=w382) -> (x-y=w381:dbl)
                n192 = Absolute Value(x=w381) -> (abs(x)=w380:dbl)
                n193 = Less Or Equal?(x=w380, y="Chival Adjust Deadband") -> (x <= y?=w378:bool)
                n194 = call-poly <vilib>:"PID.vi"("output range"="Range Chival", "PID gains"="PID Chival", "process variable"=w383, "setpoint"=w382) -> ("output"=w376:dbl)  [unwired: 6 in, 1 out]
                n195 = Select(t=Auto_Chival_Cross."Wait", s=w378, f=w388) -> (s? t:f=w387:T10)
                n196 = Negate(x=w376) -> (-x=w377:dbl)
              }
              frame "Finish" {
                n197 = global read "Robot Global Data.vi" "Auto Right"() -> (w392:dbl)
                n198 = global read "Robot Global Data.vi" "Auto Left"() -> (w391:dbl)
                n199 = global read "Robot Global Data.vi" "Reset Grayhill"() -> (w390:bool)
              }
              frame "Get NavX" {
                w396 = 0.0
                n200 = Unbundle By Name(w400) -> ("Yaw"=w407:dbl)
                n201 = global read "Robot Global Data.vi" "Auto Angle"() -> (w406:dbl)
                n202 = Increment(x=w402) -> (x+1=w401:dbl)
                n203 = Greater Or Equal?(x=w401, y=3.0) -> (x >= y?=w403:bool)
                n204 = Subtract(x=w407, y=w406) -> (x-y=w404:dbl)
                n205 = Select(t=Auto_Chival_Cross."Adjust Angle", s=w403, f=w399) -> (s? t:f=w398:T10)
                n206 = global write "Robot Global Data.vi" "Auto Angle error"(w404) -> ()
              }
              frame "Wait" {
                w408 = 0.0 ("Auto Right")
                n207 = Increment(x=w415) -> (x+1=w412:dbl)
                n208 = Greater Or Equal?(x=w412, y=5.0) -> (x >= y?=w413:bool)
                n209 = Select(t=Auto_Chival_Cross."Finish", s=w413, f=w410) -> (s? t:f=w411:T10)
              }
            }
            n210 = global write "Robot Global Data.vi" "Reset Grayhill"(w326) -> ()
            n211 = global write "Robot Global Data.vi" "Auto Crossing Finished"(w324) -> ()
            n212 = Add(x="Right Adjust speed", y=w319) -> (x+y=w317:dbl)
            n213 = Add(x=w322, y="Left Adjust speed") -> (x+y=w320:dbl)
            n214 = global write "Robot Global Data.vi" "Auto Left"(w320) -> ()
            n215 = global write "Robot Global Data.vi" "Auto Right"(w317) -> ()
          }
        }
        frame "Rough Terrain" {
          n216 = call <instrlib>:"Z900_navX_RefNum_Get.vi"("refnum name"="Navx") -> ("error out"=w416:errorcluster, "navX Device"=w417:T13)  [unwired: 9 in]
          n217 = while {
            shift-right: [w427] -> _
            shift-left: Auto_Rough_Terrain_Cross."Set NavX" -> [w434]
            tunnel: w417 -> [w433]
            tunnel: w416 -> [w432]
            shift-right: [w424] -> _
            shift-left: _ -> [w425]
            stop <- FALSE stop-if-true
            # "Go Forward the correct drift from defense"
            n218 = call <instrlib>:"Z900_navX_Get_YPRHfH.vi"("error in (no error)"=w432, "navX Device"=w433) -> ("error out"=w430:errorcluster, "YRPHfH"=w420:T2, "navX Device"=w431:T13)  [unwired: 6 in, 1 out]
            n219 = Wait (ms)(milliseconds to wait=u32 20) -> ()  [unwired: 1 out]
            n220 = case shown="\"Correct Angle\"" w434 {
              selector: w434 -> [w437 w455 w464 w480 _ w498]
              tunnel: w431 -> [w446 _ _ _ _ _]
              tunnel: w430 -> [w445 _ _ _ _ _]
              tunnel: w420 -> [w444 _ w474 w481 _ _]
              tunnel: [w443 w449 0.0 w476 w491 w494] -> w429
              tunnel: [w443 w450 0.0 w477 w492 w494] -> w428
              tunnel: [w438 w458 w465 w479 Auto_Rough_Terrain_Cross."Go to Goal" w497] -> w427
              tunnel: [TRUE _ TRUE _ w490 _] -> w426
              tunnel: w425 -> [w441 _ w469 _ _ w499]
              tunnel: [w440 _ w468 _ _ w496] -> w424
              tunnel: [_ _ _ _ TRUE ("Auto Crossing Finished") _] -> w423
              frame "Set NavX", Default {
                w443 = 0.0
                n221 = call <instrlib>:"Z900_navX_Set_ZeroYaw.vi"("error in (no error)"=w445, "navX Device"=w446) -> ()  [unwired: 8 in, 2 out]
                n222 = Unbundle By Name(w444) -> ("Yaw"=w447:dbl)
                n223 = Increment(x=w441) -> (x+1=w440:dbl)
                n224 = global write "Robot Global Data.vi" "Auto Angle"(w447) -> ()
                n225 = Greater Or Equal?(x=w440, y=3.0) -> (x >= y?=w436:bool)
                n226 = Select(t=Auto_Rough_Terrain_Cross."Go Fwd", s=w436, f=w437) -> (s? t:f=w438:T11)
              }
              frame "Go Fwd" {
                n227 = global read "Robot Global Data.vi" "Distance"() -> (w453:dbl)
                n228 = Greater Or Equal?(x=w453, y="RT 1st Distance") -> (x >= y?=w456:bool)
                n229 = Select(t=Auto_Rough_Terrain_Cross."Get Navx", s=w456, f=w455) -> (s? t:f=w458:T11)
                n230 = Greater Or Equal?(x=w453, y="RT shift speed distance") -> (x >= y?=w452:bool)
                n231 = case shown="False" w452 {
                  tunnel: ["RT 1st speed" "RT 2nd Speed"] -> w450
                  frame False {
                  }
                  frame True {
                  }
                }
                n232 = Add(x=w450, y="RT speed error") -> (x+y=w449:dbl)
              }
              frame "Get Navx" {
                n233 = Unbundle By Name(w474) -> ("Yaw"=w473:dbl)
                n234 = global read "Robot Global Data.vi" "Auto Angle"() -> (w472:dbl)
                n235 = Increment(x=w469) -> (x+1=w468:dbl)
                n236 = Greater Or Equal?(x=w468, y=50.0) -> (x >= y?=w463:bool)
                n237 = Subtract(x=w473, y=w472) -> (x-y=w466:dbl)
                n238 = Select(t=Auto_Rough_Terrain_Cross."Correct Angle", s=w463, f=w464) -> (s? t:f=w465:T11)
                n239 = global write "Robot Global Data.vi" "Auto Angle error"(w466) -> ()
              }
              frame "Correct Angle" {
                n240 = Unbundle By Name(w481) -> ("Yaw"=w487:dbl)
                n241 = global read "Robot Global Data.vi" "Auto Angle"() -> (w486:dbl)
                n242 = Subtract(x=w487, y=w486) -> (x-y=w485:dbl)
                n243 = Absolute Value(x=w485) -> (abs(x)=w484:dbl)
                n244 = Less Or Equal?(x=w484, y="RT Adjust Deadband") -> (x <= y?=w482:bool)
                n245 = call-poly <vilib>:"PID.vi"("output range"="Range RT", "PID gains"="PID RT", "process variable"=w487, "setpoint"=w486) -> ("output"=w476:dbl)  [unwired: 6 in, 1 out]
                n246 = Select(t=Auto_Rough_Terrain_Cross."Wait", s=w482, f=w480) -> (s? t:f=w479:T11)
                n247 = Negate(x=w476) -> (-x=w477:dbl)
              }
              frame "Go to Goal" {
                n248 = global read "Robot Global Data.vi" "Reset Grayhill"() -> (w490:bool)
                n249 = global read "Robot Global Data.vi" "Auto Left"() -> (w492:dbl)
                n250 = global read "Robot Global Data.vi" "Auto Right"() -> (w491:dbl)
              }
              frame "Wait" {
                w494 = 0.0 ("Auto Left")
                n251 = Increment(x=w499) -> (x+1=w496:dbl)
                n252 = Greater Or Equal?(x=w496, y=25.0) -> (x >= y?=w500:bool)
                n253 = Select(t=Auto_Rough_Terrain_Cross."Go to Goal", s=w500, f=w498) -> (s? t:f=w497:T11)
              }
            }
            n254 = global write "Robot Global Data.vi" "Auto Crossing Finished"(w423) -> ()
            n255 = global write "Robot Global Data.vi" "Auto Left"(w428) -> ()
            n256 = global write "Robot Global Data.vi" "Auto Right"(w429) -> ()
            n257 = global write "Robot Global Data.vi" "Reset Grayhill"(w426) -> ()
          }
        }
        frame "Rock Wall" {
        }
        frame "Ramparts" {
          n258 = call <instrlib>:"Z900_navX_RefNum_Get.vi"("refnum name"="Navx") -> ("error out"=w502:errorcluster, "navX Device"=w503:T13)  [unwired: 9 in]
          n259 = while {
            shift-right: [w511] -> _
            shift-left: T12."Set NavX" -> [w519]
            tunnel: w503 -> [w518]
            tunnel: w502 -> [w517]
            shift-right: [w508] -> _
            shift-left: _ -> [w509]
            stop <- w507 stop-if-true
            # "Go Forward the correct drift from defense"
            n260 = call <instrlib>:"Z900_navX_Get_YPRHfH.vi"("error in (no error)"=w517, "navX Device"=w518) -> ("error out"=w515:errorcluster, "YRPHfH"=w514:T2, "navX Device"=w516:T13)  [unwired: 6 in, 1 out]
            "YRPHfH" <- w514
            n261 = Wait (ms)(milliseconds to wait=u32 20) -> ()  [unwired: 1 out]
            n262 = case shown="\"Set NavX\", Default" w519 {
              selector: w519 -> [w521 w539 w549 w574 _]
              tunnel: w516 -> [w531 _ _ _ _]
              tunnel: w515 -> [w530 _ _ _ _]
              tunnel: w514 -> [w529 _ w559 w576 _]
              tunnel: [w528 w533 0.0 w568 w588] -> w513
              tunnel: [w528 w534 0.0 w570 w588] -> w512
              tunnel: [w522 w543 w550 w575 T12."Go to Goal" ("t")] -> w511
              tunnel: [TRUE _ TRUE _ _] -> w510
              tunnel: w509 -> [w526 _ w554 _ _]
              tunnel: [w525 _ w553 _ _] -> w508
              tunnel: [_ _ _ _ TRUE ("Auto Crossing Finished")] -> w507
              frame "Set NavX", Default {
                w528 = 0.0
                n263 = call <instrlib>:"Z900_navX_Set_ZeroYaw.vi"("error in (no error)"=w530, "navX Device"=w531) -> ()  [unwired: 8 in, 2 out]
                n264 = Unbundle By Name(w529) -> ("Yaw"=w532:dbl)
                n265 = Increment(x=w526) -> (x+1=w525:dbl)
                n266 = global write "Robot Global Data.vi" "Auto Angle"(w532) -> ()
                n267 = Greater Or Equal?(x=w525, y=3.0) -> (x >= y?=w520:bool)
                n268 = Select(t=T12."Go Fwd", s=w520, f=w521) -> (s? t:f=w522:T12)
              }
              frame "Go Fwd" {
                n269 = global read "Robot Global Data.vi" "Distance"() -> (w537:dbl)
                "encoder" <- w537
                n270 = Greater Or Equal?(x=w537, y="distancia 2") -> (x >= y?=w540:bool)
                n271 = Select(t=T12."Get Navx", s=w540, f=w539) -> (s? t:f=w543:T12)
                n272 = Greater Or Equal?(x=w537, y="Distancia 1") -> (x >= y?=w536:bool)
                n273 = case shown="False" w536 {
                  tunnel: ["velocidade 1" "velocidade 2"] -> w534
                  frame False {
                  }
                  frame True {
                  }
                }
                n274 = Add(x=w534, y="speed error") -> (x+y=w533:dbl)
              }
              frame "Get Navx" {
                n275 = Unbundle By Name(w559) -> ("Yaw"=w558:dbl)
                n276 = global read "Robot Global Data.vi" "Auto Angle"() -> (w557:dbl)
                n277 = Increment(x=w554) -> (x+1=w553:dbl)
                n278 = Greater Or Equal?(x=w553, y=3.0) -> (x >= y?=w547:bool)
                n279 = Subtract(x=w558, y=w557) -> (x-y=w551:dbl)
                "erro" <- w551
                n280 = Select(t=T12."Correct Angle", s=w547, f=w549) -> (s? t:f=w550:T12)
                n281 = global write "Robot Global Data.vi" "Auto Angle error"(w551) -> ()
              }
              frame "Correct Angle" {
                n282 = global read "Robot Global Data.vi" "Auto Angle"() -> (w565:dbl)
                "Auto Angle" <- w565
                n283 = Unbundle By Name(w576) -> ("Yaw"=w564:dbl)
                n284 = Subtract(x=w564, y=w565) -> (x-y=w566:dbl)
                n285 = Absolute Value(x=w566) -> (abs(x)=w563:dbl)
                n286 = Greater Or Equal?(x=w563, y=0.5) -> (x >= y?=w561:bool)
                "x >= y?" <- w561
                n287 = Not(x=w561) -> (.not. x?=w560:bool)
                n288 = Select(t=T12."Go to Goal", s=w560, f=w574) -> (s? t:f=w575:T12)
                n289 = global read "Robot Global Data.vi" "Auto Angle error"() -> (w572:dbl)
                n290 = case shown="True" w561 {
                  tunnel: [w583 "Adjust speed"] -> w569
                  tunnel: [w583 w584] -> w567
                  frame False {
                    w583 = 0.0
                  }
                  frame True {
                    n291 = Negate(x="Adjust speed") -> (-x=w584:dbl)
                  }
                }
                n292 = Greater Than 0?(x=w572) -> (x > 0?=w571:bool)
                n293 = case shown="False" w571 {
                  tunnel: [w578 w581] -> w570
                  tunnel: w569 -> [w579 w582]
                  tunnel: [w577 w582] -> w568
                  tunnel: w567 -> [w580 w581]
                  frame False {
                    n294 = Negate(x=w580) -> (-x=w578:dbl)
                    n295 = Negate(x=w579) -> (-x=w577:dbl)
                  }
                  frame True {
                  }
                }
              }
              frame "Go to Goal" {
                w588 = 0.0
              }
            }
            n296 = global write "Robot Global Data.vi" "Auto Left"(w512) -> ()
            n297 = global write "Robot Global Data.vi" "Auto Right"(w513) -> ()
            n298 = global write "Robot Global Data.vi" "Auto Crossing Finished"(w507) -> ()
            n299 = global write "Robot Global Data.vi" "Reset Grayhill"(w510) -> ()
          }
        }
        frame "Moat" {
        }
      }
    }
    frame Disabled {
      n300 = call <instrlib>:"Z900_navX_RefNum_Get.vi"("refnum name"="Navx") -> ("error out"=w590:errorcluster, "navX Device"=w591:T13)  [unwired: 9 in]
      n301 = while {
        shift-right: [w606] -> _
        shift-left: Auto_Porticullis_cross."Set Navx" -> [w607]
        tunnel: w591 -> [w605]
        tunnel: w590 -> [w604]
        shift-right: [w600] -> _
        shift-left: _ -> [w599]
        stop <- FALSE stop-if-true
        n302 = call <instrlib>:"Z900_navX_Get_YPRHfH.vi"("error in (no error)"=w604, "navX Device"=w605) -> ("error out"=w603:errorcluster, "YRPHfH"=w601:T2, "navX Device"=w602:T13)  [unwired: 6 in, 1 out]
        n303 = Wait (ms)(milliseconds to wait=u32 20) -> ()  [unwired: 1 out]
        n304 = case shown="\"Finish\"" w607 {
          selector: w607 -> [w616 w623 w632 w643 w652 w667 _]
          tunnel: [w617 w625 w633 w644 w651 w666 Auto_Porticullis_cross."Finish"] -> w606
          tunnel: w603 -> [w615 _ _ _ _ _ _]
          tunnel: w602 -> [w614 _ _ _ _ _ _]
          tunnel: w601 -> [w613 _ _ _ w653 w668 _]
          tunnel: [w612 _ w634 _ w654 _ _] -> w600
          tunnel: w599 -> [w611 _ w639 _ w655 _ _]
          tunnel: [w610 "Port 1st speed 2" 0.0 ("Port speed") 0.0 ("Port speed") w649 w662 w676] -> w598
          tunnel: [w610 "Port 1st speed 2" 0.0 ("Port speed") 0.0 ("Port speed") w649 w663 w677] -> w597
          tunnel: [TRUE _ TRUE w640 TRUE _ w675] -> w596
          tunnel: [_ _ _ _ _ _ TRUE] -> w594
          frame "Set Navx", Default {
            w610 = 0.0
            n305 = call <instrlib>:"Z900_navX_Set_ZeroYaw.vi"("error in (no error)"=w615, "navX Device"=w614) -> ()  [unwired: 8 in, 2 out]
            n306 = Unbundle By Name(w613) -> ("Yaw"=w620:dbl)
            n307 = Increment(x=w611) -> (x+1=w612:dbl)
            n308 = global write "Robot Global Data.vi" "Auto Angle"(w620) -> ()
            n309 = Greater Or Equal?(x=w612, y=3.0) -> (x >= y?=w618:bool)
            n310 = Select(t=Auto_Porticullis_cross."Adjust angle", s=w618, f=w616) -> (s? t:f=w617:T9)
          }
          frame "Go Fwd" {
            n311 = global write "Robot Global Data.vi" "B Button"(TRUE ("B Button")) -> ()
            n312 = global read "Robot Global Data.vi" "Distance"() -> (w627:dbl)
            n313 = Greater Or Equal?(x=w627, y="Port 1st Distance 2") -> (x >= y?=w624:bool)
            n314 = Select(t=Auto_Porticullis_cross."Cross Porticullis", s=w624, f=w623) -> (s? t:f=w625:T9)
          }
          frame "Wait 1" {
            n315 = global write "Robot Global Data.vi" "B Button"(FALSE ("B Button")) -> ()
            n316 = Increment(x=w639) -> (x+1=w634:dbl)
            n317 = Greater Or Equal?(x=w634, y=30.0) -> (x >= y?=w635:bool)
            n318 = Select(t=Auto_Porticullis_cross."Cross Porticullis", s=w635, f=w632) -> (s? t:f=w633:T9)
          }
          frame "Cross Porticullis" {
            n319 = global write "Robot Global Data.vi" "Start Button"(TRUE ("Start Button")) -> ()
            n320 = global read "Robot Global Data.vi" "Finished Porticullis crossing"() -> (w642:bool)
            n321 = Select(t=Auto_Porticullis_cross."Get Navx", s=w642, f=w643) -> (s? t:f=w644:T9)
            n322 = global read "Robot Global Data.vi" "Reset Grayhill"() -> (w640:bool)
          }
          frame "Get Navx" {
            w649 = 0.0
            n323 = Unbundle By Name(w653) -> ("Yaw"=w660:dbl)
            n324 = global read "Robot Global Data.vi" "Auto Angle"() -> (w659:dbl)
            n325 = Increment(x=w655) -> (x+1=w654:dbl)
            n326 = Greater Or Equal?(x=w654, y=3.0) -> (x >= y?=w656:bool)
            n327 = Subtract(x=w660, y=w659) -> (x-y=w657:dbl)
            n328 = Select(t=Auto_Porticullis_cross."Adjust angle", s=w656, f=w652) -> (s? t:f=w651:T9)
            n329 = global write "Robot Global Data.vi" "Auto Angle error"(w657) -> ()
          }
          frame "Adjust angle" {
            n330 = Unbundle By Name(w668) -> ("Yaw"=w672:dbl)
            "Yaw" <- w672
            n331 = Subtract(x=w672, y="Angle Setpoint") -> (x-y=w671:dbl)
            n332 = Absolute Value(x=w671) -> (abs(x)=w670:dbl)
            n333 = Less Or Equal?(x=w670, y=3.0) -> (x <= y?=w669:bool)
            n334 = call-poly <vilib>:"PID.vi"("output range"="Range Port 2", "PID gains"="PID Port 2", "process variable"=w672, "setpoint"="Angle Setpoint") -> ("output"=w663:dbl)  [unwired: 6 in, 1 out]
            n335 = Select(t=Auto_Porticullis_cross."Finish", s=w669, f=w667) -> (s? t:f=w666:T9)
            n336 = Negate(x=w663) -> (-x=w662:dbl)
          }
          frame "Finish" {
            n337 = global read "Robot Global Data.vi" "Reset Grayhill"() -> (w675:bool)
            n338 = global read "Robot Global Data.vi" "Auto Right"() -> (w677:dbl)
            n339 = global read "Robot Global Data.vi" "Auto Left"() -> (w676:dbl)
          }
        }
        n340 = global write "Robot Global Data.vi" "Auto Right"(w597) -> ()
        n341 = global write "Robot Global Data.vi" "Auto Left"(w598) -> ()
        n342 = global write "Robot Global Data.vi" "Reset Grayhill"(w596) -> ()
        n343 = global write "Robot Global Data.vi" "Auto Crossing Finished"(w594) -> ()
      }
    }
  }
